vi "GetType.vi"(8 "error in (no error)":errorcluster, 11 "Configure AM Enabled [AM] Msg":refnum<class "Configure AM Enabled [AM] Msg.lvclass">) -> (0 "error out":errorcluster, 2 "Data Sample":variant, 3 "Configure AM Enabled [AM] Msg":refnum<class "Configure AM Enabled [AM] Msg.lvclass">)   [LabVIEW 2016, in "CS++Fgen.lvlib" / "Configure AM Enabled [AM] Msg.lvclass"]
doc: "This VI delivers a sample of the data type format the message expects."
uses:
  Configure AM Enabled [AM] Msg.lvclass
  Configure AM Enabled [AM] Msg.lvclass/Configure AM Enabled [AM] Msg.ctl
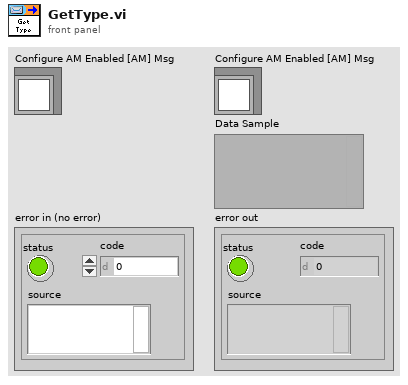
[diagram p1: front panel]
types:
  T1 = cluster{"Channel Name (\"\")":string, "AM enabled (True)":bool}
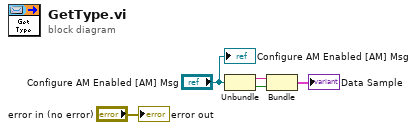
[diagram p0: block diagram]
diagram:
  n1 = Unbundle("Configure AM Enabled [AM] Msg") -> (w2:string, w1:bool)
  n2 = Bundle("Channel Name (\"\")"=w2, "AM enabled (True)"=w1) -> (→"Data Sample":T1)  [unwired: 1 in]
  "error out" <- "error in (no error)"
  "Configure AM Enabled [AM] Msg" <- "Configure AM Enabled [AM] Msg"
